vi "Create_ID.vi"(1 "ID Argument Name":string, 2 "Input Sequence":cluster{string, string[], dbl[], dbl}[](array[cluster])) -> (0 "ID":string)   [LabVIEW 2011]
doc: "This VI finds an unused ID (integer >= 1) in the sequence and returns it as a string."
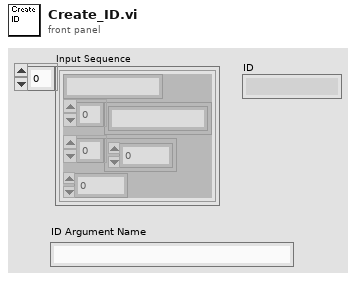
[diagram p1: front panel]
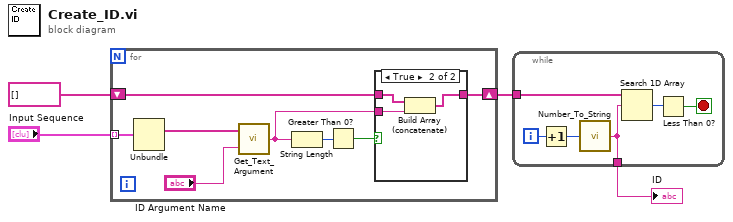
[diagram p0: block diagram]
diagram:
  n1 = for {
    tunnel: "Input Sequence" -> [w12] mode=indexing
    shift-right: [w8] -> w2
    shift-left: string[] [] -> [w7]
    n2 = Unbundle(w12) -> (w11:string[])  [unwired: 3 out]
    n3 = call "Get_Text_Argument.vi"("Argument"="ID Argument Name", "Argument List"=w11) -> ("Text"=w9:string)
    n4 = String Length(string=w9) -> (length=w10:i32)
    n5 = Greater Than 0?(x=w10) -> (x > 0?=w6:bool)
    n6 = case shown="True" w6 {
      tunnel: w9 -> [_ w16]
      tunnel: [w13 w15] -> w8
      tunnel: w7 -> [w13 w14]
      frame False {
      }
      frame True {
        n7 = Build Array (concatenate)(w14, w16) -> (w15:string[])
      }
    }
  }
  n8 = while {
    tunnel: w2 -> [w21]
    tunnel: [w17] -> w1
    i -> [w22]
    stop <- w19 stop-if-true
    n9 = Increment(x=w22) -> (x+1=w18:i32)
    n10 = call "Number_To_String.vi"("Number"=w18) -> ("String"=w17:string)
    n11 = Search 1D Array(1D array=w21, element=w17) -> (index of element=w20:i32)  [unwired: 1 in]
    n12 = Less Than 0?(x=w20) -> (x < 0?=w19:bool)
  }
  "ID" <- w1
